vi "Thorlabs General File IO Module.vi"(4 "Data Range":T1={"Z start (pxl)"=0, "Z length (pxl)"=400}, 5 "Data In":sgl[][](array[numeric]), 6 "Imaging Parameters":T2, 7 "Actions":enum16{"Create", "Write", "Write Data", "Close"}(ring)=enum."Write Data", 8 "error in":errorcluster, 9 "Scan Parameters":T3={"# Scan"={"#Ascan"=400, "#Bscan"=400}, "# Rpt"={"#ARpt"=1, "#BRpt"=1}, "Aline Rate"=2, "# Extra"={"# ARpt_extra"=5, "#Brtn_extra"=60}} {"Aline Rate" items=["76 KHz", "146 KHz", "76 KHz", "28 KHz", "10 KHz"]}, 10 "Raw Data In":u16[][](array[numeric]), 11 "Save Path":path=path "E:/Jiarui/1217test") -> (0 "error out":errorcluster, 2 "Scan Parameter":string, 3 "Save Name":string)   [LabVIEW 2017]
panel:
  out "subarray":u16[](graph)
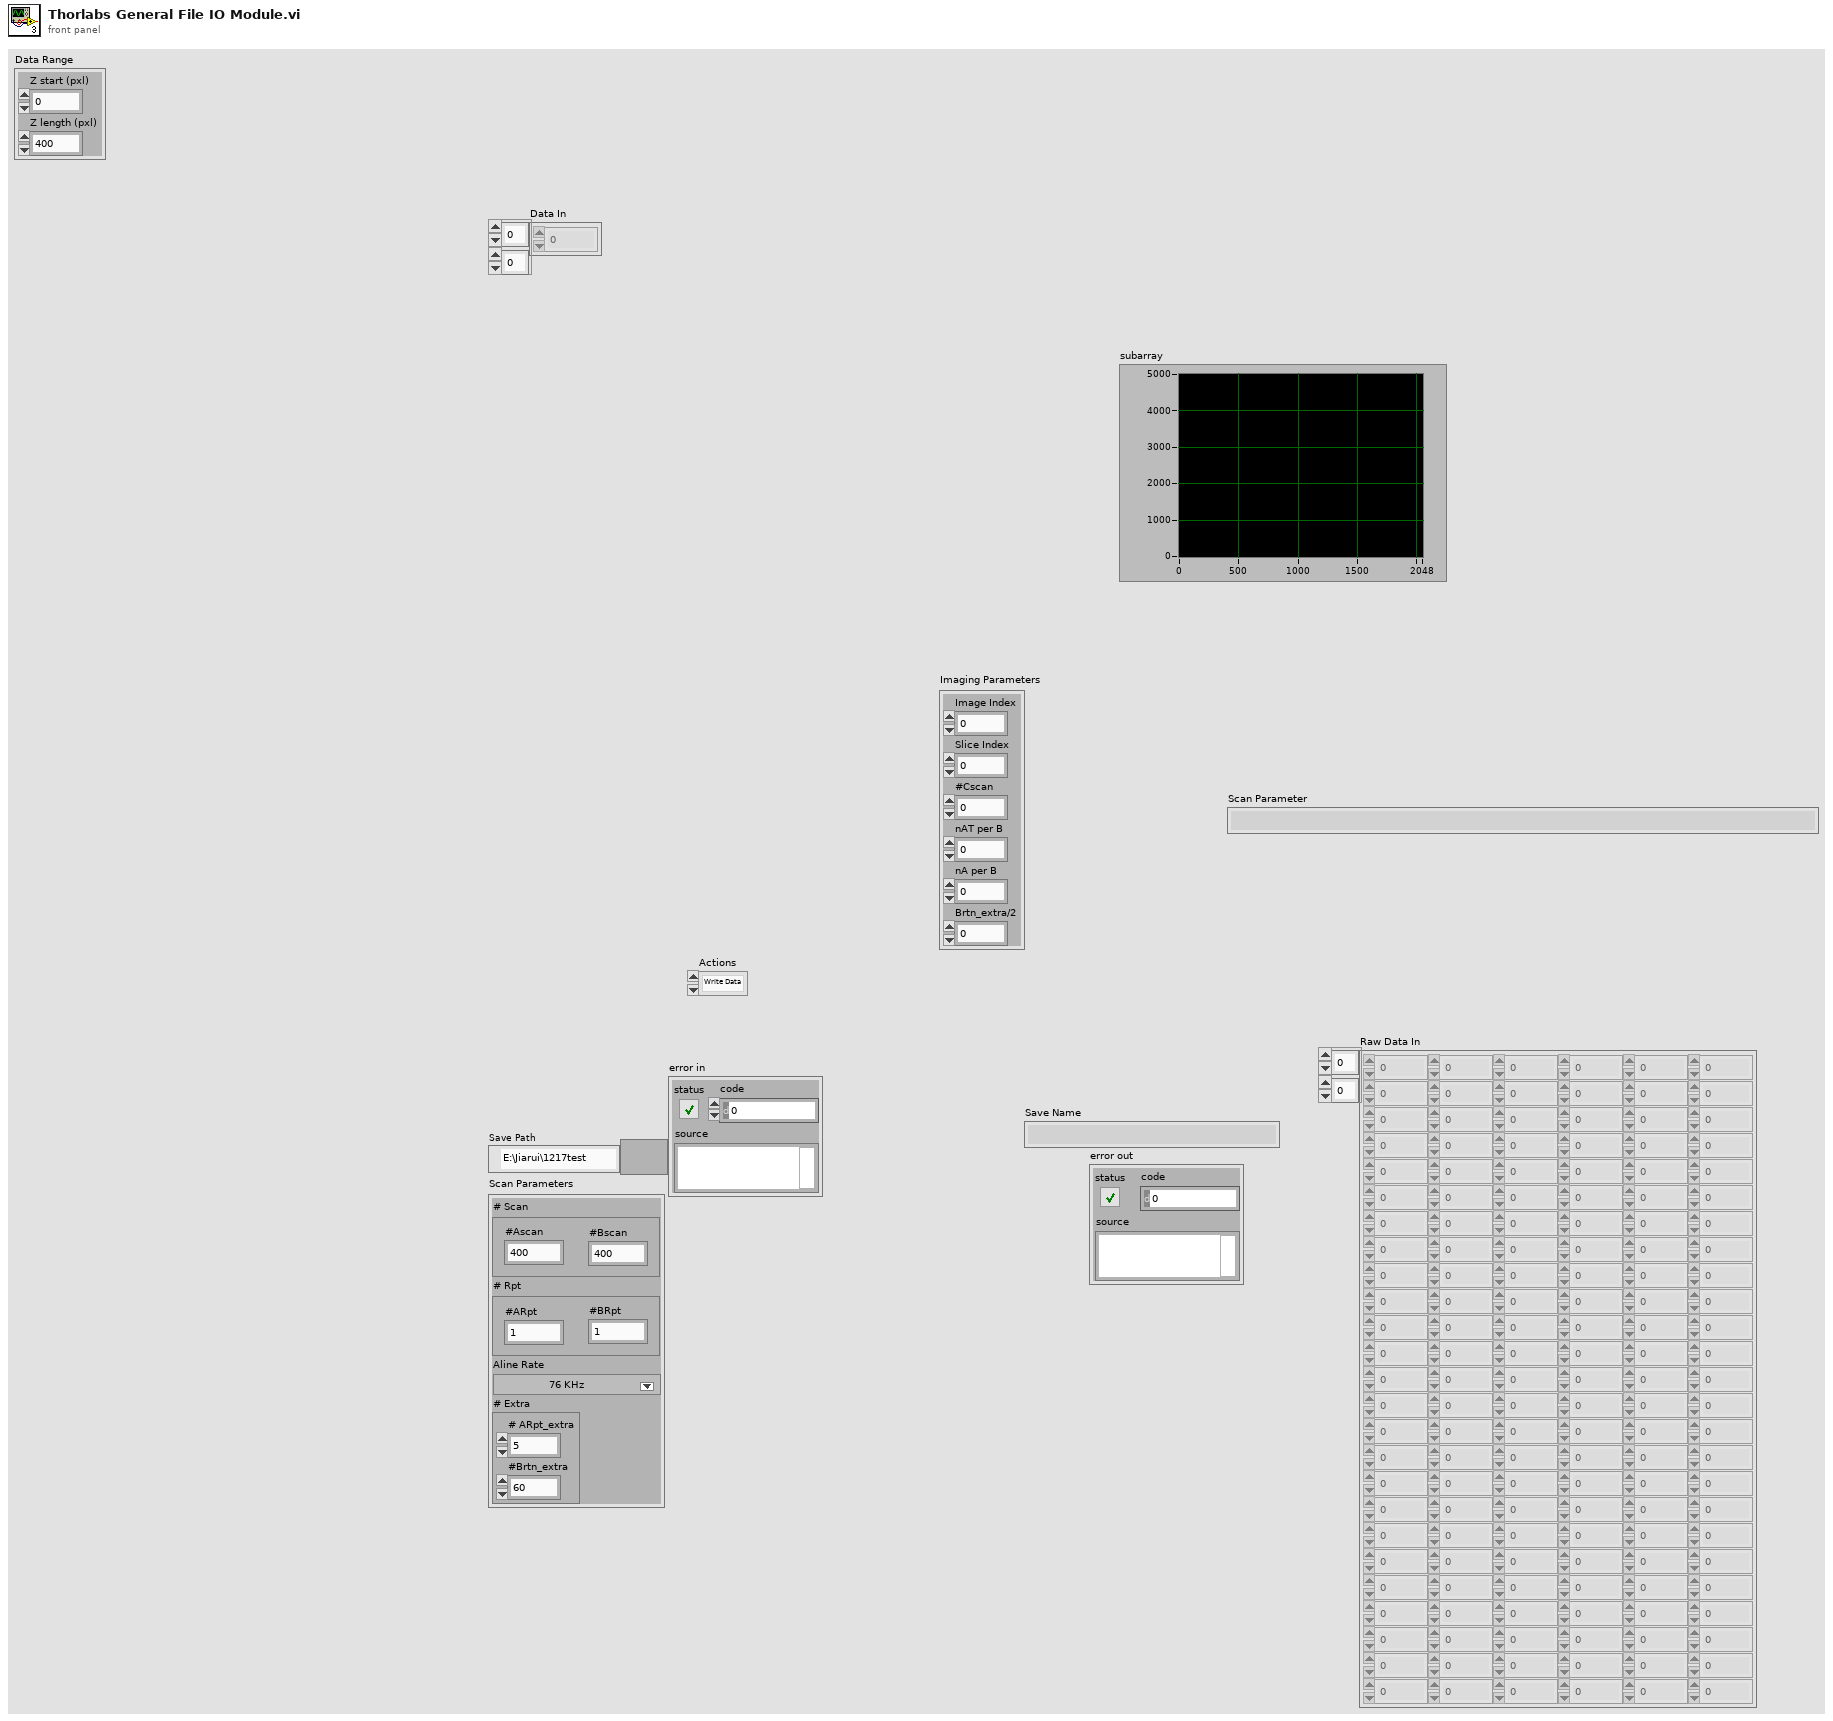
[diagram p1: front panel]
types:
  T1 = cluster{"Z start (pxl)":i32, "Z length (pxl)":i32}
  T2 = cluster{"Image Index":i16, "Slice Index":i16, "#Cscan":i32, "nAT per B":i32, "nA per B":i32, "Brtn_extra/2":i32}
  T3 = cluster{"# Scan":cluster{"#Ascan":i32, "#Bscan":i32}, "# Rpt":cluster{"#ARpt":i32, "#BRpt":i32}, "Aline Rate":u16, "# Extra":cluster{"# ARpt_extra":i32, "#Brtn_extra":i32}}
  T4 = enum16{"open", "replace", "create", "open or create", "replace or create", "replace or create with confirmation"}
  T5 = enum16{"big-endian, network order", "native, host order", "little-endian"}
  T6 = cluster{"nAT per B":i32, "Brtn_extra/2":i32, "nA per B":i32}
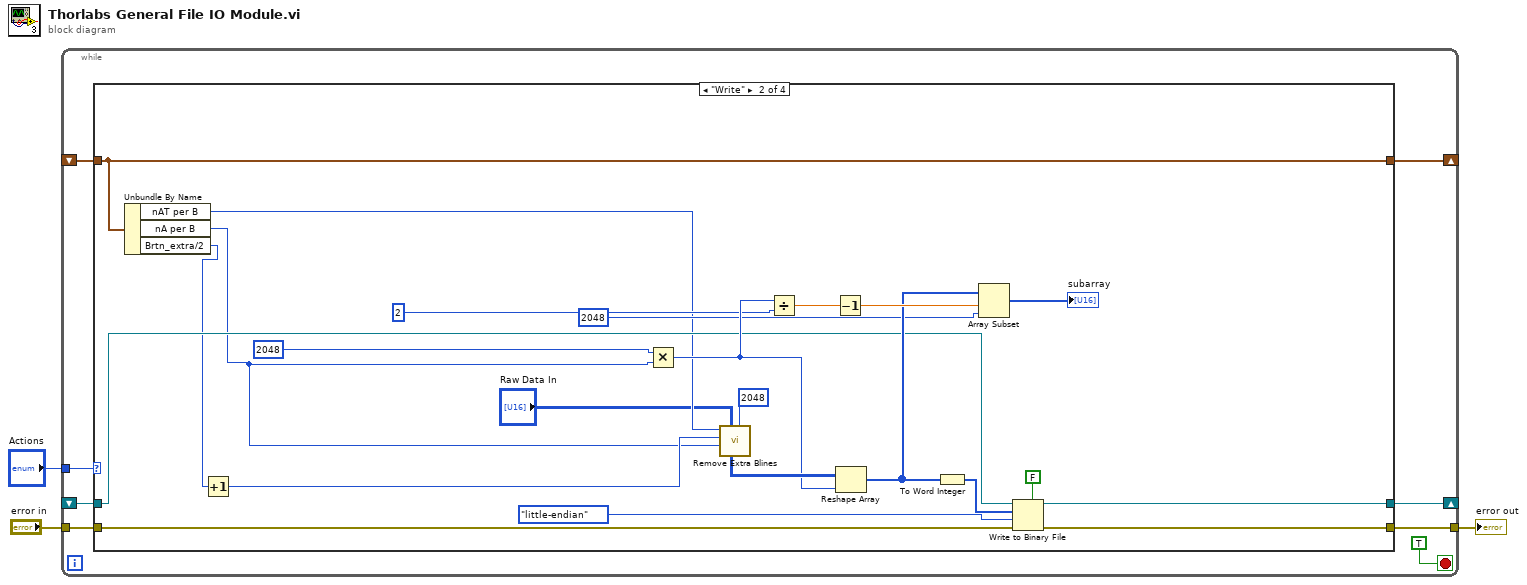
[diagram p0: block diagram]
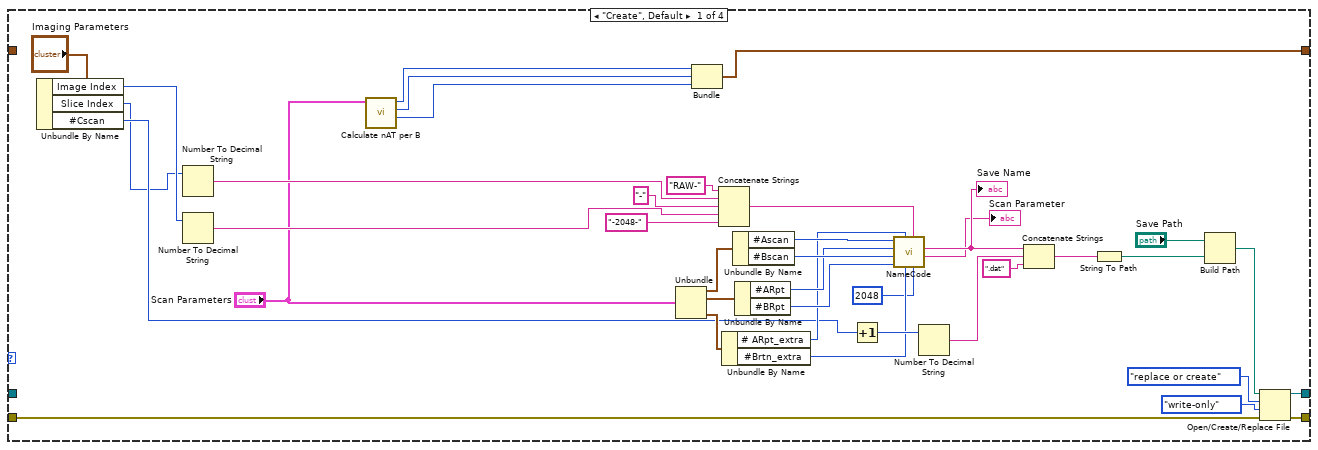
[diagram p2: hidden frame]
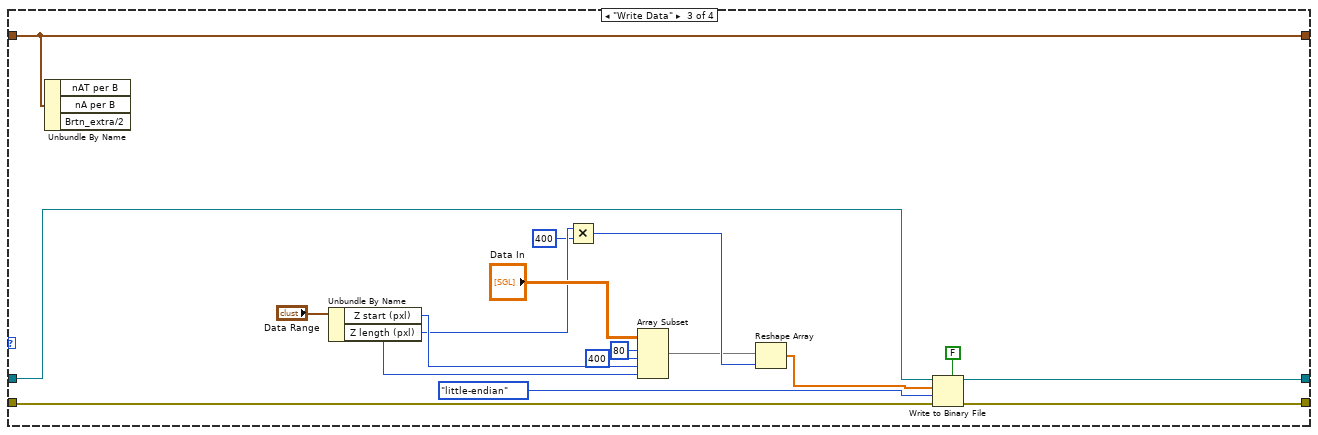
[diagram p3: hidden frame]
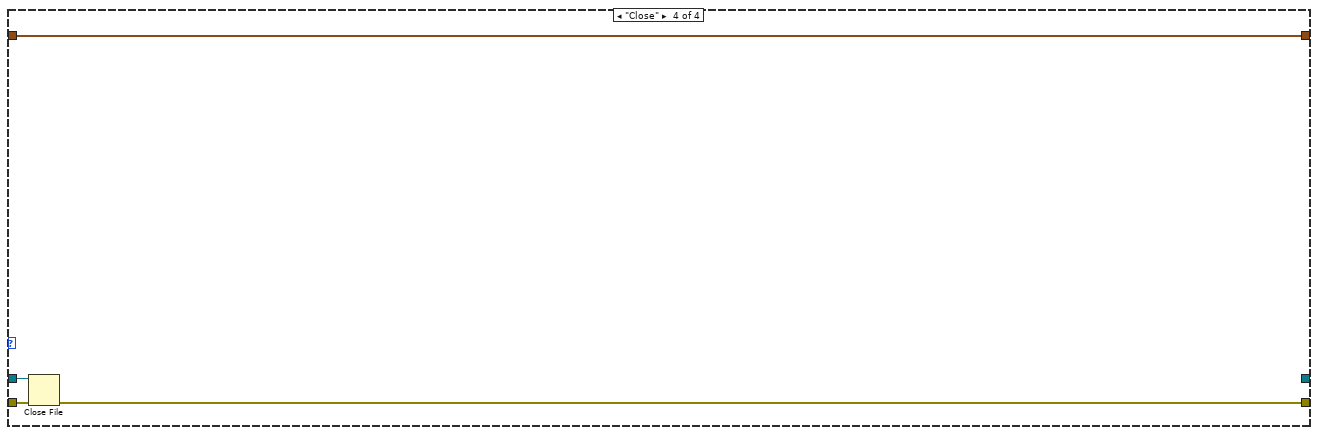
[diagram p4: hidden frame]
diagram:
  n1 = while {
    tunnel: "Actions" -> [w10]
    tunnel: "error in" -> [w9]
    tunnel: [w8] -> w1
    shift-right: [w7] -> _
    shift-left: _ -> [w6]
    shift-right: [w5] -> _
    shift-left: _ -> [w4]
    stop <- TRUE stop-if-true
    n2 = case shown="\"Write\"" w10 {
      tunnel: w9 -> [w21 w57 w87 w94]
      tunnel: [w22 w58 w88 w92] -> w8
      tunnel: [w23 w59 w86 _] -> w7
      tunnel: w6 -> [_ w60 w84 w93]
      tunnel: [w12 w56 w85 w91] -> w5
      tunnel: w4 -> [_ w56 w85 w91]
      frame "Create", Default {
        n3 = Unbundle By Name("Imaging Parameters") -> ("Image Index"=w19:i16, "Slice Index"=w18:i16, "#Cscan"=w20:i32)
        n4 = Number To Decimal String(number=w18) -> (decimal integer string=w32:string)  [unwired: 1 in]
        n5 = Number To Decimal String(number=w19) -> (decimal integer string=w33:string)  [unwired: 1 in]
        n6 = call "Calculate nAT per B.vi"("Scan Parameters"="Scan Parameters") -> ("nA per B"=w13:i32, "Brtn_extra/2"=w14:i32, "nAT per B"=w15:i32)  [unwired: 8 in]
        n7 = Unbundle("Scan Parameters") -> ("# Scan"=w31:cluster{"#Ascan":i32, "#Bscan":i32}, "# Rpt"=w35:cluster{"#ARpt":i32, "#BRpt":i32}, "# Extra"=w36:cluster{"# ARpt_extra":i32, "#Brtn_extra":i32})  [unwired: 1 out]
        n8 = Bundle("nAT per B"=w15, "Brtn_extra/2"=w14, "nA per B"=w13) -> (w12:T6)  [unwired: 1 in]
        n9 = Concatenate Strings("RAW-" ("Name0"), w32, "-" ("string"), w33, "-2048-" ("string")) -> (w34:string)
        n10 = Unbundle By Name(w36) -> ("# ARpt_extra"=w37:i32, "#Brtn_extra"=w38:i32)
        n11 = Unbundle By Name(w31) -> ("#Ascan"=w40:i32, "#Bscan"=w42:i32)
        n12 = Unbundle By Name(w35) -> ("#ARpt"=w41:i32, "#BRpt"=w43:i32)
        n13 = Increment(x=w20) -> (x+1=w47:i32)
        n14 = call "NameCode.vi"("# Z"=2048, "Name0"=w34, "# BRtn extra"=w38, "# ARpt extra"=w37, "# B rpt"=w43, "# B scan"=w42, "# A rpt"=w41, "# Aline"=w40) -> ("Scan Parameter"=→"Scan Parameter":string, "Name Code"=w48:string)  [unwired: 2 in]
        "Save Name" <- w48
        n15 = Number To Decimal String(number=w47) -> (decimal integer string=w46:string)  [unwired: 1 in]
        n16 = Concatenate Strings(w48, w46, ".dat" ("string")) -> (w45:string)
        n17 = String To Path(string=w45) -> (path=w44:path)
        n18 = Build Path(base path="Save Path", name or relative path=w44) -> (appended path=w50:path)
        n19 = Open/Create/Replace File(file path (use dialog)=w50, error in=w21, operation (0:open)=T4."replace or create", access (0:read/write)=enum16{"read/write", "read-only", "write-only"}."write-only") -> (refnum out=w23:refnum<file>, error out=w22:errorcluster)  [unwired: 2 in, 1 out]
      }
      frame "Write" {
        n20 = Unbundle By Name(w56) -> ("nAT per B"=w54:i32, "nA per B"=w55:i32, "Brtn_extra/2"=w53:i32)
        n21 = Increment(x=w53) -> (x+1=w73:i32)
        n22 = Multiply(x=2048 ("dimension size"), y=w55) -> (x*y=w69:i32)
        n23 = call "Remove Extra Blines.vi"("Z size (pxl)"=2048, "Data In"="Raw Data In", "#Aline"=w55, "Start index"=w73, "nAT per B"=w54) -> ("Data Out"=w72:u16[][])  [unwired: 6 in]
        n24 = Divide(x=w69, y=2) -> (x/y=w70:dbl)
        n25 = Decrement(x=w70) -> (x-1=w71:dbl)
        n26 = Reshape Array(w72, w69) -> (w67:u16[])
        n27 = To Word Integer(number=w67) -> (16bit integer=w66:i16[])
        n28 = Array Subset(array=w67, index=w71, length=2048) -> (→"subarray":u16[])
        n29 = Write to Binary File(file (use dialog)=w60, data=w66, error in=w57, 5:FALSE ("prepend array or string size? (T)"), 9:T5."little-endian" ("byte order (0:big-endian, network order)")) -> (refnum out=w59:refnum<file>, error out=w58:errorcluster)  [unwired: 1 in, 1 out]
      }
      frame "Write Data" {
        n30 = Unbundle By Name(w85) -> ()  [unwired: 3 out]
        n31 = Unbundle By Name("Data Range") -> ("Z start (pxl)"=w79:i32, "Z length (pxl)"=w78:i32)
        n32 = Multiply(x=w78, y=400) -> (x*y=w83:i32)
        n33 = Array Subset(array="Data In", index (row)=80 ("index"), length (row)=400 ("length"), index (col)=w79, length (col)=w78) -> (w81:sgl[][])
        n34 = Reshape Array(w81, w83) -> (w77:sgl[])
        n35 = Write to Binary File(file (use dialog)=w84, data=w77, error in=w87, 5:FALSE ("prepend array or string size? (T)"), 9:T5."little-endian" ("byte order (0:big-endian, network order)")) -> (refnum out=w86:refnum<file>, error out=w88:errorcluster)  [unwired: 1 in, 1 out]
      }
      frame "Close" {
        n36 = Close File(refnum=w93, error in=w94) -> (error out=w92:errorcluster)  [unwired: 1 out]
      }
    }
  }
  "error out" <- w1
